vi "SubVI_DriveBackwards_Auto.vi"(0 "False = Encoders average True = Encoders reading seperately":bool, 1 "Inches to target":dbl=-18.85 format="%#_13g", 2 "Speed":dbl=-3000.0, 4 "PIDF":dbl[](array[numeric])) -> ()   [LabVIEW 2017]
uses:
  <vilib>/Rock Robotics/WPI/ThirdParty/Phoenix-LabVIEW/Motor Controller/Controls/CTRE_Phoenix_MotorControl_ControlMode.ctl
  <vilib>/Rock Robotics/WPI/ThirdParty/Phoenix-LabVIEW/Motor Controller/Get/CTRE_Phoenix_MotorController_GetSelectedSensorData.vi
panel:
  out "Encoder Average":dbl
  out "Position(Left encoder)":dbl
  out "Position(Right encoder)":dbl
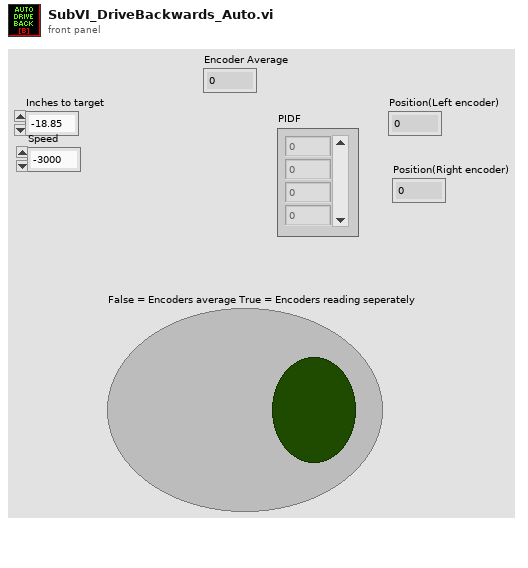
[diagram p1: front panel]
types:
  T1 = typedef "WPI_MotorControlDeviceRef.ctl" = cluster{"DeviceStatus":errorcluster, "Type":T2, "PWM":cluster{"PWM Channel":T3, "DeadBand":T4}, "CAN":cluster{"Device Number":u8, "SetOutput VI Ref":variant, "GetOutput VI Ref":variant, "Enable VI Ref":variant, "Disable VI Ref":variant, "Data":variant}, "Invert":bool, "DIO PWM":cluster{"PWM \"Enable\" Channel":T3, "DIOChannel":T5, "PWM Rate":dbl}}
  T2 = typedef "WPI_MotorControlType.ctl" = enum16{"PWM", "CAN", "DIO PWM"}
  T3 = typedef "FPGA_DIOPWMChannel.ctl" = enum8{"PWM 0", "PWM 1", "PWM 2", "PWM 3", "PWM 4", "PWM 5", "PWM 6", "PWM 7", "PWM 8", "PWM 9", "PWM MXP 0", "PWM MXP 1", "PWM MXP 2", "PWM MXP 3", "PWM MXP 4", "PWM MXP 5", "PWM MXP 6", "PWM MXP 7", "PWM MXP 8", "PWM MXP 9", "Invalid"}
  T4 = typedef "WPI_PWMDeadband.ctl" = cluster{"Name":string, "maxPositivePwm":i32, "minPositivePwm":i32, "centerPwm":i32, "maxNegativePwm":i32, "minNegativePwm":i32, "angularRange":u16}
  T5 = typedef "FPGA_DIOChannel.ctl" = enum8{"DIO 0", "DIO 1", "DIO 2", "DIO 3", "DIO 4", "DIO 5", "DIO 6", "DIO 7", "DIO 8", "DIO 9", "DIO MXP 0", "DIO MXP 1", "DIO MXP 2", "DIO MXP 3", "DIO MXP 4", "DIO MXP 5", "DIO MXP 6", "DIO MXP 7", "DIO MXP 8", "DIO MXP 9", "DIO MXP 10", "DIO MXP 11", "DIO MXP 12", "DIO MXP 13", "DIO MXP 14", "DIO MXP 15", "SPI Port CS1", "SPI Port CS2", "SPI Port CS3", "SPI Port MISO", "SPI Port MOSI", "Invalid"}
  T6 = typedef "CTRE_Phoenix_MotorControl_ControlMode.ctl" = u16
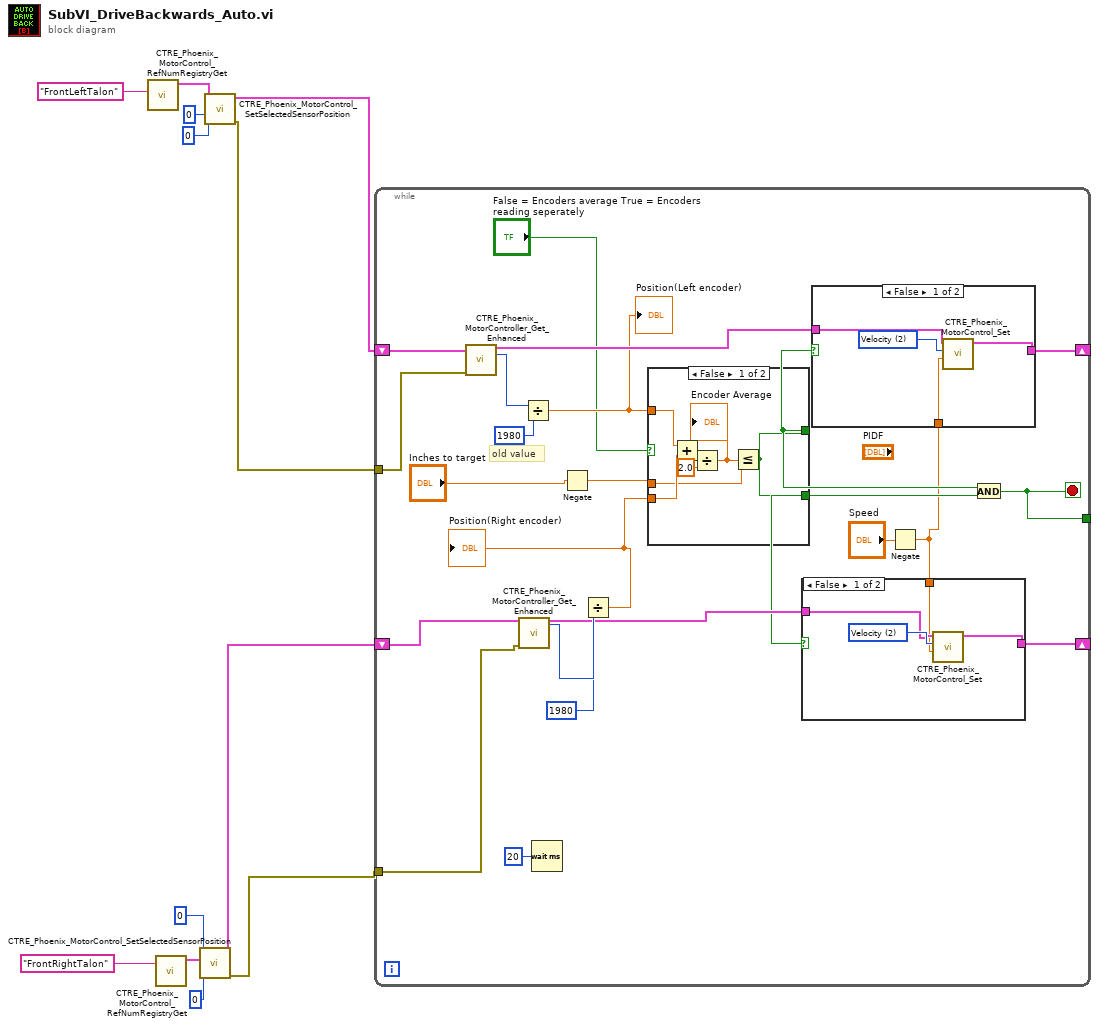
[diagram p0: block diagram]
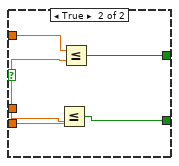
[diagram p2: hidden frame]
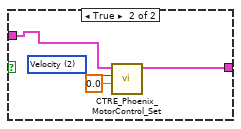
[diagram p3: hidden frame]
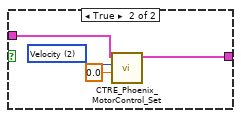
[diagram p4: hidden frame]
diagram:
  n1 = call <vilib>:"CTRE_Phoenix_MotorControl_RefNumRegistryGet.vi"("refnum name"="FrontLeftTalon") -> ("PhoenixMotorControlDevRef"=w4:T1)  [unwired: 9 in, 1 out]
  n2 = call <vilib>:"CTRE_Phoenix_MotorControl_RefNumRegistryGet.vi"("refnum name"="FrontRightTalon") -> ("PhoenixMotorControlDevRef"=w8:T1)  [unwired: 9 in, 1 out]
  n3 = call <vilib>:"CTRE_Phoenix_MotorControl_SetSelectedSensorPosition.vi"("pidLoopIdx"=u32 0, "New Sensor Position"=0, "PhoenixMotorControlDevRef"=w8) -> ("error out"=w2:errorcluster, "PhoenixMotorControlDevRef"=w5:T1)  [unwired: 7 in]
  n4 = call <vilib>:"CTRE_Phoenix_MotorControl_SetSelectedSensorPosition.vi"("pidLoopIdx"=u32 0, "New Sensor Position"=0, "PhoenixMotorControlDevRef"=w4) -> ("error out"=w1:errorcluster, "PhoenixMotorControlDevRef"=w3:T1)  [unwired: 7 in]
  n5 = while {
    shift-right: [w32] -> _
    shift-left: w3 -> [w31]
    shift-right: [w30] -> _
    shift-left: w5 -> [w27]
    tunnel: [w15] -> _
    tunnel: w2 -> [w13]
    tunnel: w1 -> [w14]
    stop <- w15 stop-if-true
    # "old value"
    n6 = call-poly <vilib>:"CTRE_Phoenix_MotorController_Get_Enhanced.vi"("PhoenixMotorControlDevRef"=w31, "error in"=w14) -> ("PhoenixMotorControlDevRef"=w33:T1, "Position (Raw Sensor Units)"=w35:i32)  [unwired: 10 in, 2 out]
    n7 = call-poly <vilib>:"CTRE_Phoenix_MotorController_Get_Enhanced.vi"("PhoenixMotorControlDevRef"=w27, "error in"=w13) -> ("PhoenixMotorControlDevRef"=w26:T1, "Position (Raw Sensor Units)"=w28:i32)  [unwired: 10 in, 2 out]
    n8 = Divide(x=w35, y=1980) -> (x/y=w24:dbl)
    "Position(Left encoder)" <- w24
    n9 = Wait (ms)(milliseconds to wait=u32 20) -> ()  [unwired: 1 out]
    n10 = Negate(x="Inches to target") -> (-x=w18:dbl)
    n11 = Divide(x=w28, y=1980) -> (x/y=w23:dbl)
    "Position(Right encoder)" <- w23
    n12 = case shown="False" "False = Encoders average True = Encoders reading seperately" {
      tunnel: w24 -> [w42 w47]
      tunnel: w23 -> [w41 w46]
      tunnel: w18 -> [w38 w45]
      tunnel: [w37 w44] -> w22
      tunnel: [w37 w43] -> w21
      frame False {
        n13 = Add(x=w42, y=w41) -> (x+y=w40:dbl)
        n14 = Divide(x=w40, y=2.0) -> (x/y=w39:dbl)
        "Encoder Average" <- w39
        n15 = Less Or Equal?(x=w39, y=w38) -> (x <= y?=w37:bool)
      }
      frame True {
        n16 = Less Or Equal?(x=w46, y=w45) -> (x <= y?=w43:bool)
        n17 = Less Or Equal?(x=w47, y=w45) -> (x <= y?=w44:bool)
      }
    }
    n18 = Negate(x="Speed") -> (-x=w16:dbl)
    n19 = case shown="False" w21 {
      tunnel: [w50 w53] -> w30
      tunnel: w26 -> [w49 w52]
      tunnel: w16 -> [w48 _]
      frame False {
        w51 = T6 2 items=["PercentOutput"=0, "Position"=1, "Velocity"=2, "Current"=3, "Follower"=5, "MotionProfile"=6, "MotionMagic"=7, "MotionMagicArc"=8, "MotionProfileArc"=10, "Disabled"=15] ("Control Mode")
        n20 = call <vilib>:"CTRE_Phoenix_MotorControl_Set.vi"("Output"=w48, "Control Mode"=w51, "PhoenixMotorControlDevRef"=w49) -> ("PhoenixMotorControlDevRef"=w50:T1)  [unwired: 7 in, 1 out]
      }
      frame True {
        w54 = T6 2 items=["PercentOutput"=0, "Position"=1, "Velocity"=2, "Current"=3, "Follower"=5, "MotionProfile"=6, "MotionMagic"=7, "MotionMagicArc"=8, "MotionProfileArc"=10, "Disabled"=15] ("Control Mode")
        n21 = call <vilib>:"CTRE_Phoenix_MotorControl_Set.vi"("Output"=0.0, "Control Mode"=w54, "PhoenixMotorControlDevRef"=w52) -> ("PhoenixMotorControlDevRef"=w53:T1)  [unwired: 7 in, 1 out]
      }
    }
    n22 = case shown="False" w22 {
      tunnel: w33 -> [w58 w63]
      tunnel: [w57 w60] -> w32
      tunnel: w16 -> [w56 _]
      frame False {
        w59 = T6 2 items=["PercentOutput"=0, "Position"=1, "Velocity"=2, "Current"=3, "Follower"=5, "MotionProfile"=6, "MotionMagic"=7, "MotionMagicArc"=8, "MotionProfileArc"=10, "Disabled"=15] ("Control Mode")
        n23 = call <vilib>:"CTRE_Phoenix_MotorControl_Set.vi"("Output"=w56, "Control Mode"=w59, "PhoenixMotorControlDevRef"=w58) -> ("PhoenixMotorControlDevRef"=w57:T1)  [unwired: 7 in, 1 out]
      }
      frame True {
        w61 = T6 2 items=["PercentOutput"=0, "Position"=1, "Velocity"=2, "Current"=3, "Follower"=5, "MotionProfile"=6, "MotionMagic"=7, "MotionMagicArc"=8, "MotionProfileArc"=10, "Disabled"=15] ("Control Mode")
        n24 = call <vilib>:"CTRE_Phoenix_MotorControl_Set.vi"("Output"=0.0, "Control Mode"=w61, "PhoenixMotorControlDevRef"=w63) -> ("PhoenixMotorControlDevRef"=w60:T1)  [unwired: 7 in, 1 out]
      }
    }
    n25 = And(x=w22, y=w21) -> (x .and. y?=w15:bool)
  }
